vi "Measurement Logic.vi"() -> ()   [LabVIEW 2021, in "Crosstalk Sweep.lvlib"]
uses:
  Crosstalk Sweep.lvlib
  Measurement Configuration.ctl
  shared/controls/digital output level units.ctl
  shared/controls/sweep profile.ctl
  shared/controls/weighting filter.ctl
  shared/controls/highpass filter.ctl
  shared/controls/lowpass filter.ctl
  Measurement Results.ctl
  <vilib>/MeasurementLink/MeasurementLink Measurement Server/Measure Call Context/Measure Call Context.lvclass
  shared/controls/audio filter settings.ctl
  <vilib>/Analysis/1siggen.llb/Ramp Pattern by Samples.vi
  <vilib>/addons/_NISVFA/_Shared subVIs/Common/SVL Set dB Reference (N Ch - 1 Ref).vi
  <vilib>/addons/_NISVFA/_Spectrum Processing/SVFA Unit Conversion (Complex) (N Ch).vi
  <vilib>/addons/_NISVFA/_Spectrum Processing/SVFA Unit Conversion (Complex) (1 Ch).vi
  <vilib>/addons/_NISVFA/_Shared subVIs/Common/SVL Set dB Reference (1 Ch).vi
  <vilib>/addons/_NISVFA/_Shared subVIs/Common/svc_Log View for Spectrum (1Ch).vi
  <vilib>/addons/_NISVFA/_Spectrum Processing/SVFA Unit Conversion (1 Ch).vi
  <vilib>/addons/_NISVFA/_Shared subVIs/Common/svc_Complex Datatype Defaults.vi
  <vilib>/addons/_NISVFA/_Shared subVIs/Common/SVL Set dB Reference (variant).vi
  <vilib>/addons/_NISVFA/_Shared subVIs/Common/svc_Unwrap Phase.vi
  <vilib>/addons/_NISVFA/_Shared subVIs/Common/svc_Convert Spectrum Array to dB.vi
  <vilib>/addons/_NISVFA/_Shared subVIs/Common/svc_Spectrum Units.vi
  <vilib>/addons/_NISVFA/_Spectrum Processing/subVIs/svfa_Conversion Utility (spectrum info).vi
  <vilib>/addons/_NISVFA/_Shared subVIs/Common/svc_Format Value (DBL).vi
  <vilib>/addons/_NISVFA/_Shared subVIs/Common/svc_Get Weighting Enum and Labels.vi
  <vilib>/addons/_NISVFA/_Shared subVIs/Common/svc_Engineering Units to Unit Label.vi
  <vilib>/addons/_NISVFA/_Shared subVIs/Common/svc_Surround NonAlpha String with Parentheses.vi
  <vilib>/dlg_ctls.llb/Space Constant.vi
  <vilib>/addons/_NISVFA/_Spectrum Processing/subVIs/svfa_Peak to RMS to Peak2Peak.vi
  <vilib>/addons/_NISVFA/_Spectrum Processing/subVIs/svfa_Mag to Mag2.vi
  <vilib>/addons/_NISVFA/_Spectrum Processing/subVIs/svfa_Linear to dB.vi
  <vilib>/addons/_NISVFA/_Spectrum Processing/subVIs/svfa_dBrefA to dBrefB.vi
  <vilib>/addons/_NISVFA/_Spectrum Processing/subVIs/svfa_Spectrum to Spectral Density.vi
  <vilib>/addons/_NISVFA/_Shared subVIs/Common/svc_Unit Label Lexical Class.vi
  <vilib>/addons/_NISVFA/_Shared subVIs/Common/svc_Window Parameters.vi
  <vilib>/DAQmx/create/channels.llb/DAQmx Create Channel (AI-Voltage-Basic).vi
  <vilib>/DAQmx/configure/timing.llb/DAQmx Timing (Sample Clock).vi
  <vilib>/Waveform/WDTOps.llb/WDT Get Waveform Subset DBL.vi
  <vilib>/addons/_NISVFA/_Shared subVIs/Common/svc_Caller VI Returned in Error Source.vi
  <vilib>/Analysis/4window.llb/window parameters.vi
  <vilib>/Analysis/4window.llb/Window Properties.vi
  <vilib>/Analysis/4window.llb/Window Properties by Name.vi
  <vilib>/Analysis/NI_AALBase.lvlib
  shared/digital serial api/Digital Serial.lvclass
  shared/digital serial gen settings/digital audio protocol controls.lvlib
  shared/controls/audio controls.lvlib
panel:
  out "XY Graph":cluster{"X data":dbl[], "Y data":dbl[]}[](graph)=[{"X data"=[1000.0000079066498, 1444.4445068435625, 1888.8885404873877, 2333.332974551163, 2777.7776191924368, 3222.2221837594147, 3666.6669921625667, 4111.111180056958, 4555.555303242544, 5000.000080001889], "Y data"=[-83.02077381288392, -79.93403033517882, -79.67645242718531, -75.93201157658373, -75.45566870671045, -74.17335893170335, -72.78173878108285, -72.07408908843989, -70.96339966107612, -70.06311639272025]}, {"X data"=[1000.0000079066498, 1444.4445068435625, 1888.8885404873877, 2333.332974551163, 2777.7776191924368, 3222.2221837594147, 3666.6669921625667, 4111.111180056958, 4555.555303242544, 5000.000080001889], "Y data"=[-100.3560709729349, -100.71622632785073, -100.77370759881723, -100.70292296094586, -100.93312934835308, -99.69443859013792, -100.53907016781393, -100.4790465149002, -101.0239883463542, -100.13211237211175]}, {"X data"=[1000.0000079066498, 1444.4445068435625, 1888.8885404873877, 2333.332974551163, 2777.7776191924368, 3222.2221837594147, 3666.6669921625667, 4111.111180056958, 4555.555303242544, 5000.000080001889], "Y data"=[-117.76654421705797, -127.52260822953843, -128.9925376198278, -120.72766654102435, -118.4793948341033, -122.29285627461928, -135.7344906838366, -121.41325998155511, -120.01195459277108, -131.15607832666257]}]
  out "Spectrum":cluster{"x0":dbl, "dx":dbl, "magnitude":dbl[]}[](graph)
  out "Waveform Graph":waveform(dbl)[](graph)
  out "measure call context out":refnum<class "Measure Call Context.lvclass">
  in  "measure call context in":refnum<class "Measure Call Context.lvclass">
  out "measurement results":T1={"channel names"=["PXI1Slot4/ai0", "PXI1Slot4/ai1", "PXI1Slot2/ai0", "PXI1Slot2/ai1"], "frequency (Hz)"=[1000.0000079066498, 1444.4445068435625, 1888.8885404873877, 2333.332974551163, 2777.7776191924368, 3222.2221837594147, 3666.6669921625667, 4111.111180056958, 4555.555303242544, 5000.000080001889], "crosstalk (dB)"=[-83.02077381288392, -79.93403033517882, -79.67645242718531, -75.93201157658373, -75.45566870671045, -74.17335893170335, -72.78173878108285, -72.07408908843989, -70.96339966107612, -70.06311639272025, -100.3560709729349, -100.71622632785073, -100.77370759881723, -100.70292296094586, -100.93312934835308, -99.69443859013792, -100.53907016781393, -100.4790465149002, -101.0239883463542, -100.13211237211175, -117.76654421705797, -127.52260822953843, -128.9925376198278, -120.72766654102435, -118.4793948341033, -122.29285627461928, -135.7344906838366, -121.41325998155511, -120.01195459277108, -131.15607832666257], "wfm - t0"=0.0, "wfm - dt"=1.9531249997269942e-05, "wfm - data"=array[20480 elements], "fft - f0"=0.0, "fft - df"=10.00000000139779, "fft - data"=array[10240 elements]}
  in  "measurement configuration":T2={"digital serial cfg file"="C:\\Users\\SEBUADV\\Desktop\\Jack\\TAS6424.dsgcfg", "digital channel list"="7821\\PCMo 8", "master clock channel list"="7821\\PCMo 0", "digital audio interferrer channel"=0, "output level"=10.0, "output level units"=enum."% FS", "output range (pk-pk)"=15.0, "load impedance"=4.0, "acq channel - victim"="PXI1Slot4/ai1, PXI1Slot2/ai0:1", "acq channel - interferrer"="PXI1Slot4/ai0", "acq sampling rate"=51200.0, "sweep start frequency (Hz)"=1000.0, "sweep stop frequency (Hz)"=5000.0, "number of steps"=10, "sweep profile"=enum."Linear", "min measurement cycles"=20, "min measurement time (s)"=0.1, "min settling cycles"=0, "min settling time (s)"=0.005, "weighting filter"=enum."Linear", "highpass filter"=enum."DC", "lowpass filter"=enum."No filter"} {"min measurement time (s)" format="%0.2f"; "acq sampling rate" format="%0.2f"}
  out "error out":errorcluster
  in  "error in":errorcluster
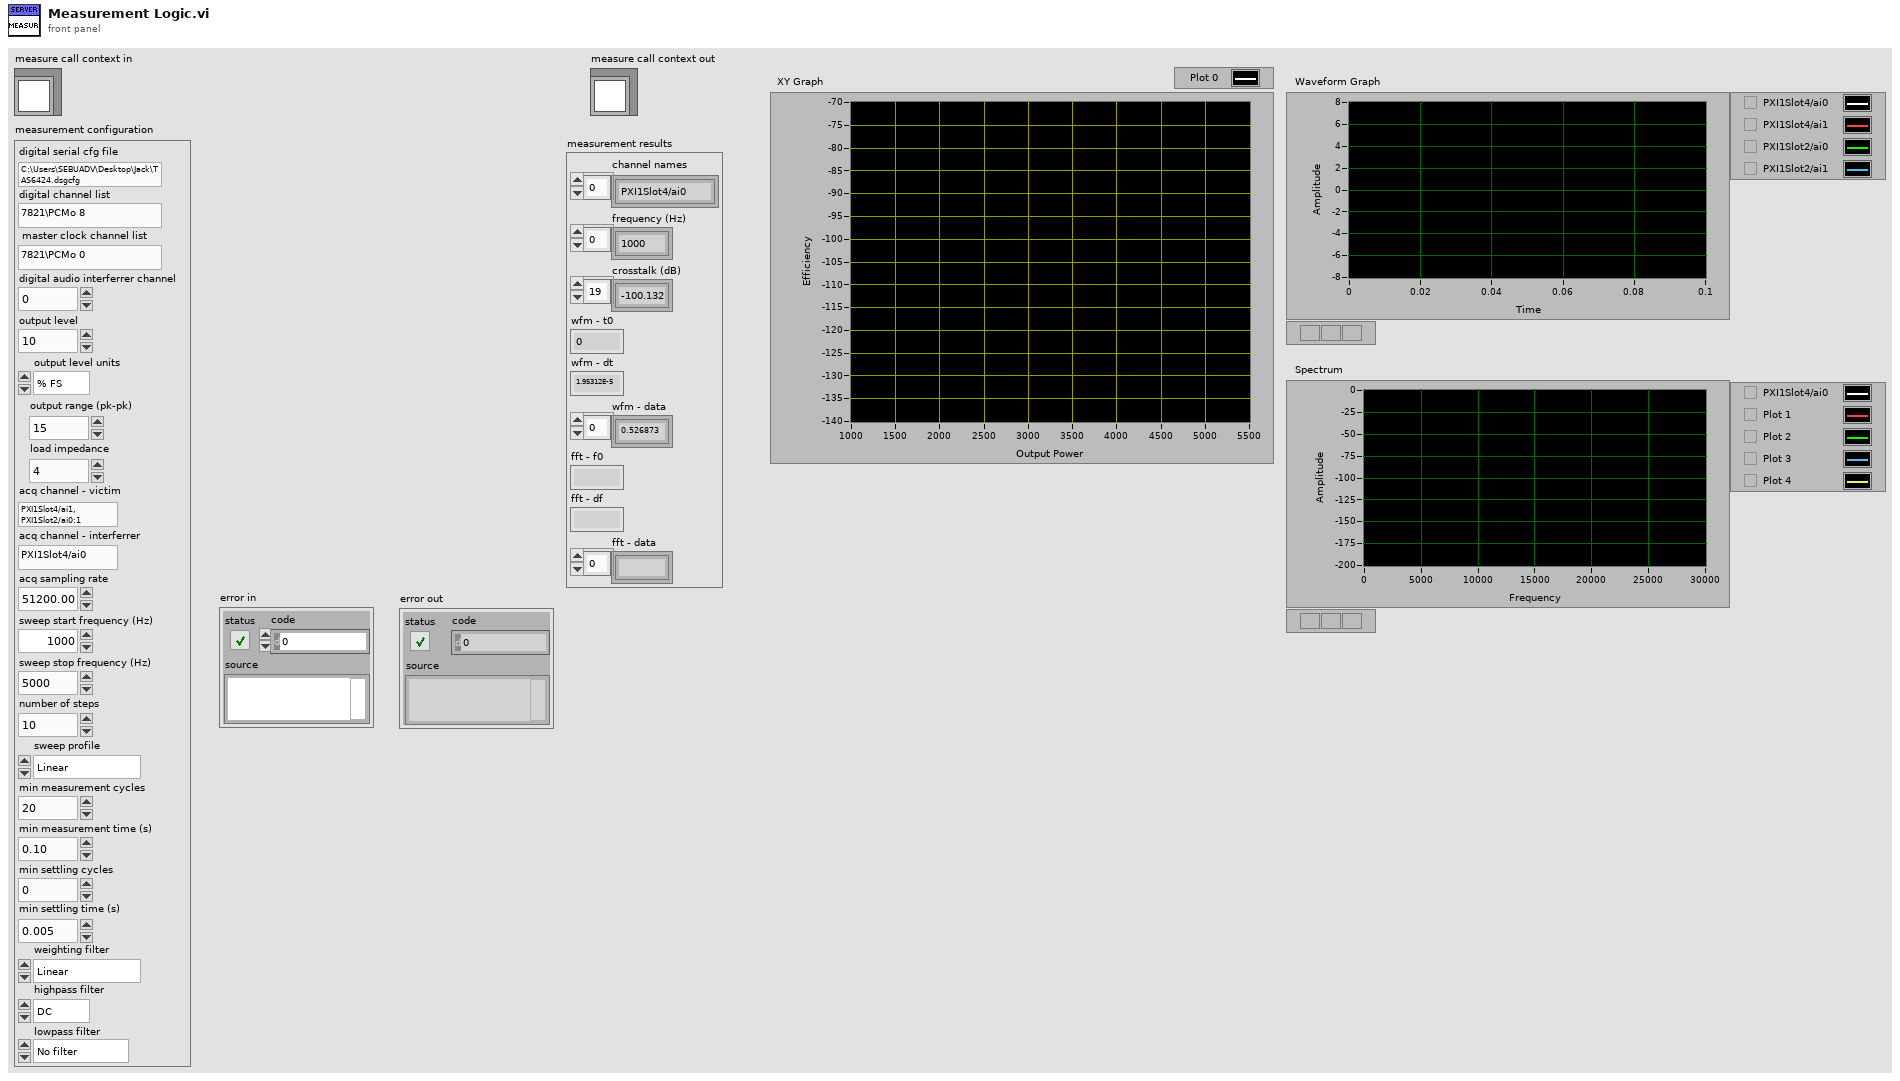
[diagram p1: front panel]
types:
  T1 = typedef "Crosstalk Sweep.lvlib/Measurement Results.ctl" = cluster{"channel names":string[], "frequency (Hz)":dbl[], "crosstalk (dB)":dbl[], "wfm - t0":dbl, "wfm - dt":dbl, "wfm - data":dbl[], "fft - f0":dbl, "fft - df":dbl, "fft - data":dbl[]}
  T2 = typedef "Crosstalk Sweep.lvlib/Measurement Configuration.ctl" = cluster{"digital serial cfg file":string, "digital channel list":string, "master clock channel list":string, "digital audio interferrer channel":i32, "output level":dbl, "output level units":T3, "output range (pk-pk)":dbl, "load impedance":dbl, "acq channel - victim":string, "acq channel - interferrer":string, "acq sampling rate":dbl, "sweep start frequency (Hz)":dbl, "sweep stop frequency (Hz)":dbl, "number of steps":u32, "sweep profile":T4, "min measurement cycles":u32, "min measurement time (s)":dbl, "min settling cycles":u32, "min settling time (s)":dbl, "weighting filter":T5, "highpass filter":T6, "lowpass filter":T7}
  T3 = typedef "audio controls.lvlib/digital output level units.ctl" = enum32{"% FS", "dBFS", "V"}
  T4 = typedef "audio controls.lvlib/sweep profile.ctl" = enum32{"Linear", "Logarithmic"}
  T5 = typedef "weighting filter.ctl" = enum32{"Linear", "A-weighting", "B-weighting", "C-weighting"}
  T6 = typedef "highpass filter.ctl" = enum32{"DC", "AC"}
  T7 = typedef "lowpass filter.ctl" = enum32{"No filter", "AES17 20kHz", "AES17 40kHz"}
  T8 = typedef "audio filter settings.ctl" = cluster{"weighting filter":T5, "highpass filter":T6, "lowpass filter ":T7}
  T9 = typedef "digital serial gen settings.ctl" = cluster{"number of channels":u32, "data justification":T10, "endianness":T11, "channel length":u32, "bit depth":u32, "frame clock rate":dbl, "bit clock edge sync":T12, "master clock rate":dbl, "Logic Level":T13, "frame sync edge for channel 0":T12, "Channel 0 Offset":u32}
  T10 = typedef "PDM Shared.lvlib/PCM Data Justification.ctl" = enum16{"Left Justified", "Right Justified"}
  T11 = typedef "PDM Shared.lvlib/PCM Bit Endianness.ctl" = enum16{"MSB First", "LSB First"}
  T12 = typedef "PDM Shared.lvlib/Digital Edge.ctl" = enum8{"Rising", "Falling"}
  T13 = typedef "PDM Acquisition Class Library.lvlib/DecoderSession.lvclass/Logic Levels.ctl" = enum16{"3.3 V", "1.8 V", "1.2 V"}
  T14 = typedef "AudioGenTypeDefs.lvlib/digital protocol settings.ctl" = cluster{"logic level":T13, "PCM Data Configuration":T15, "bit clock rate":sgl, "master clock rate":sgl, "clock mode":T16, "Frame Sync Clock Control":T17}
  T15 = typedef "PDM Shared.lvlib/PCM Data Format Configuration.ctl" = cluster{"Frame Sync Edge for Channel 0":T12, "Channel Count Per Frame":u8, "Channel Length":u16, "Bit Depth":u8, "Channel 0 Offset":u16, "Endianness":T11, "Data Justification":T10}
  T16 = typedef "PDM Shared.lvlib/clock mode.ctl" = enum16{"divided clock", "DDS"}
  T17 = typedef "PDM Shared.lvlib/PCM Frame Sync Control.ctl" = cluster{"Frame Length":u16, "Frame Sync Pulse Width":u16, "Bit Clock Edge  Sync":T12}
  T18 = cluster{"frequency":dbl, "amplitude":dbl, "phase":dbl}[]
  T19 = cluster{"linear/dB":enum16{"no change", "linear", "dB"}, "dB reference (0: no change)":dbl, "power/magnitude":enum16{"no change", "power", "magnitude"}, "view":enum16{"no change", "rms", "peak", "peak-peak"}}
  T20 = typedef "svc_Spectrum Info.ctl" = cluster{"channel name":string, "description":string, "x-axis units":T21, "spectral info":cluster{"spectrum type":T22, "linear/dB":enum16{"linear", "dB"}, "window":u16, "window size":i32, "FFT size":i32}, "engineering units":T23, "custom label":string, "dB reference [EU]":dbl, "peak units":enum16{"rms", "peak", "peak-peak"}, "weighting filter":T24, "spectral density?":bool, "unit label":string, "spectrum skewed?":bool, "complimentary spectrum units":T25}
  T21 = typedef "svc_X-Axis Units.ctl" = u16
  T22 = typedef "svc_Spectrum Type.ctl" = enum16{"FFT Spectrum [complex]", "Amplitude [Magnitude]", "Power [Magnitude^2]", "Cross Spectrum [complex]", "Frequency Response [Complex]"}
  T23 = typedef "svc_Engineering Units Text Ring.ctl" = u16
  T24 = typedef "svc_Weighting Filter Text Ring.ctl" = u16
  T25 = typedef "svc_Complimentary Spectrum Units.ctl" = enum16{"none", "radians", "degrees", "cycles", "imaginary"}
  T26 = cluster{"complex spectrum response":cluster{"f0":dbl, "df":dbl, "complex spectrum":cdb[]}, "spectrum info":T20}
  T27 = cluster{"complex spectrum response":cluster{"f0":dbl, "df":dbl, "complex spectrum":cdb[]}, "spectrum info":T20}[]
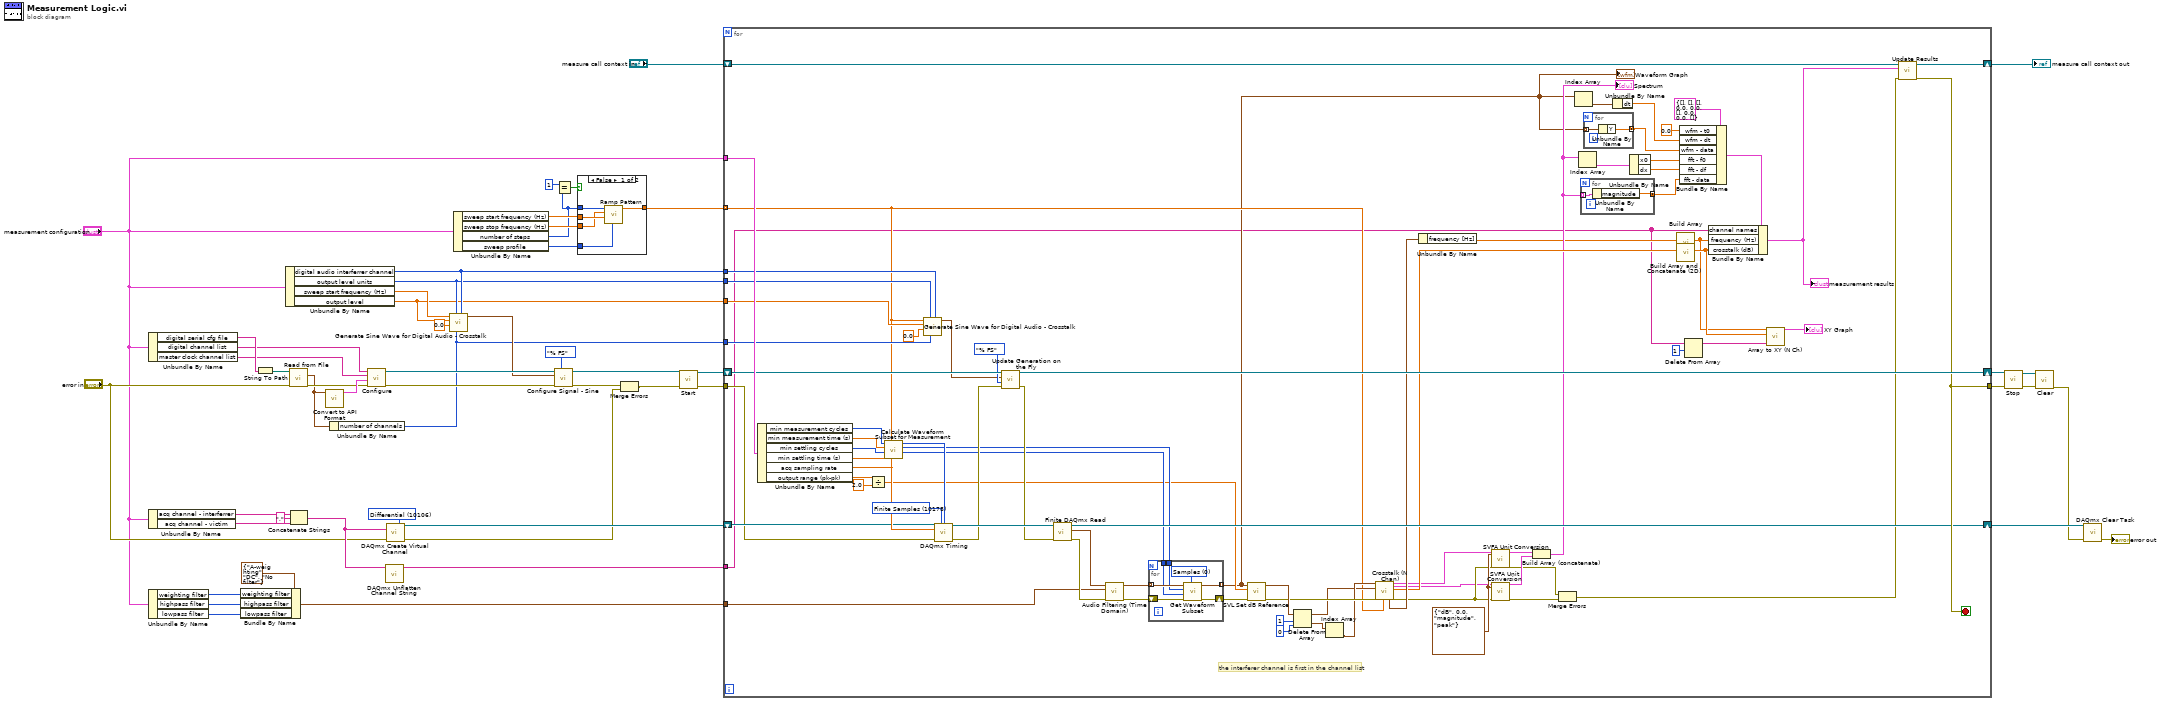
[diagram p0: block diagram]
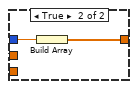
[diagram p2: hidden frame]
diagram:
  w28 = 10106 items=["Default"=-1, "RSE"=10083, "NRSE"=10078, "Differential"=10106, "Pseudodifferential"=12529] ("input terminal configuration")
  n1 = Unbundle By Name("measurement configuration") -> ("digital serial cfg file"=w44:string, "digital channel list"=w40:string, "master clock channel list"=w39:string)
  n2 = Unbundle By Name("measurement configuration") -> ("acq channel - interferrer"=w27:string, "acq channel - victim"=w26:string)
  n3 = Unbundle By Name("measurement configuration") -> ("weighting filter"=w4:T5, "highpass filter"=w3:T6, "lowpass filter"=w2:T7)
  n4 = Bundle By Name(cluster=T8 {"weighting filter"=enum."A-weighting", "highpass filter"=enum."DC", "lowpass filter "=enum."No filter"} ("filter settings"), "weighting filter"=w4, "highpass filter"=w3, "lowpass filter"=w2) -> (w1:T8)
  n5 = String To Path(string=w44) -> (path=w41:path)
  n6 = Unbundle By Name("measurement configuration") -> ("digital audio interferrer channel"=w17:i32, "output level units"=w16:T3, "sweep start frequency (Hz)"=w31:dbl, "output level"=w15:dbl)
  n7 = call "Read from File.vi"("error in (no error)"="error in", "file path"=w41) -> ("error out"=w42:errorcluster, "digital audio protocol settings"=w33:T9)  [unwired: 7 in, 1 out]
  n8 = Concatenate Strings(w27, "," ("string"), w26) -> (w24:string)
  n9 = call "Convert to API Format.vi"("digital audio protocol settings"=w33) -> ("digital protocol settings"=w43:T14)  [unwired: 10 in]
  n10 = Unbundle By Name(w33) -> ("number of channels"=w14:u32)
  n11 = call "Configure.vi"("error in (no error)"=w42, "digital protocol settings"=w43, "master clock channel list"=w39, "data channel list"=w40) -> ("error out"=w38:errorcluster, "digital serial task"=w37:refnum<class "Digital Serial.lvclass">)  [unwired: 6 in]
  n12 = call <vilib>:"DAQmx Unflatten Channel String.vi"("names in"=w24) -> ("names out"=w18:string[])  [unwired: 13 in, 1 out]
  n13 = call-poly <vilib>:"DAQmx Create Virtual Channel.vi"("input terminal configuration"=w28, "physical channels"=w24, "error in"="error in") -> ("task out"=w20:refnum<k21>, "error out"=w19:errorcluster)  [unwired: 11 in]
  n14 = call "Generate Sine Wave for Digital Audio - Crosstalk.vi"("interferrer channel"=w17, "number of channels"=w14, "output level units"=w16, "phase"=0.0, "amplitude"=w15, "frequency"=w31) -> ("signals"=w32:T18)  [unwired: 5 in]
  n15 = Unbundle By Name("measurement configuration") -> ("sweep start frequency (Hz)"=w50:dbl, "sweep stop frequency (Hz)"=w49:dbl, "number of steps"=w47:u32, "sweep profile"=w51:T4)
  n16 = call "Configure Signal - Sine.vi"("output level units"=digital_output_level_units."% FS", "error in (no error)"=w38, "sine wave properties"=w32, "Digital Serial in"=w37) -> ("error out"=w35:errorcluster, "Digital Serial out"=w36:refnum<class "Digital Serial.lvclass">)  [unwired: 6 in]
  n17 = Equal?(x=u32 1, y=w47) -> (x = y?=w48:bool)
  n18 = case shown="False" w48 {
    tunnel: w51 -> [w58 _]
    tunnel: w50 -> [w57 w60]
    tunnel: w49 -> [w56 _]
    tunnel: w47 -> [w55 _]
    tunnel: [w54 w59] -> w45
    frame False {
      n19 = call-poly <vilib>:"Ramp Pattern.vi"("type"=w58, "start"=w57, "end"=w56, "samples"=w55) -> ("Ramp Pattern"=w54:dbl[])  [unwired: 6 in, 1 out]
    }
    frame True {
      n20 = Build Array(w60) -> (w59:dbl[])
    }
  }
  n21 = Merge Errors(w35, w19) -> (w34:errorcluster)
  n22 = call "Start.vi"("error in (no error)"=w34, "Digital Serial in"=w36) -> ("error out"=w21:errorcluster, "Digital Serial out"=w22:refnum<class "Digital Serial.lvclass">)  [unwired: 8 in]
  n23 = for {
    tunnel: w45 -> [w86] mode=indexing
    shift-right: [w136] -> w53
    shift-left: "measure call context in" -> [w135]
    shift-right: [w105] -> w9
    shift-left: w20 -> [w121]
    shift-right: [w107] -> w11
    shift-left: w22 -> [w116]
    tunnel: w21 -> [w120]
    tunnel: "measurement configuration" -> [w119]
    tunnel: w18 -> [w64]
    tunnel: w17 -> [w114]
    tunnel: w16 -> [w113]
    tunnel: w15 -> [w111]
    tunnel: w14 -> [w110]
    tunnel: [w106] -> w10
    tunnel: w1 -> [w100]
    stop <- w106 stop-if-true
    w83 = T19 {"linear/dB"=enum."dB", "dB reference (0: no change)"=0.0, "power/magnitude"=enum."magnitude", "view"=enum."peak"} ("desired scaling")
    w123 = 10178 items=["Finite Samples"=10178, "Continuous Samples"=10123, "Hardware Timed Single Point"=12522] ("sample mode")
    # "the interferer channel is first in the channel list"
    n24 = Unbundle By Name(w119) -> ("min measurement cycles"=w128:u32, "min measurement time (s)"=w127:dbl, "min settling cycles"=w126:u32, "min settling time (s)"=w125:dbl, "acq sampling rate"=w122:dbl, "output range (pk-pk)"=w95:dbl)
    n25 = Divide(x=w95, y=2.0) -> (x/y=w94:dbl)
    n26 = call "Calculate Waveform Subset for Measurement.vi"("sampling rate"=w122, "signal frequency"=w86, "minimum settling duration"=w125, "minimum settling cycles"=w126, "minimum measurement duration"=w127, "minimum measurement cycles"=w128) -> ("duration (samples)"=w98:u32, "start (samples)"=w99:u32, "total acquisition (samples)"=w124:u32)  [unwired: 3 in]
    n27 = call "Generate Sine Wave for Digital Audio - Crosstalk.vi"("interferrer channel"=w114, "number of channels"=w110, "output level units"=w113, "phase"=0.0, "amplitude"=w111, "frequency"=w86) -> ("signals"=w109:T18)  [unwired: 5 in]
    n28 = call-poly <vilib>:"DAQmx Timing.vi"("task/channels in"=w121, "sample mode"=w123, "samples per channel"=w124, "rate"=w122, "error in"=w120) -> ("task out"=w118:refnum<k21>, "error out"=w117:errorcluster)  [unwired: 9 in]
    n29 = call "Update Generation on the Fly.vi"("error in (no error)"=w117, "output level units"=digital_output_level_units."% FS", "sine wave properties"=w109, "Digital Serial in"=w116) -> ("error out"=w108:errorcluster, "Digital Serial out"=w107:refnum<class "Digital Serial.lvclass">)  [unwired: 6 in]
    n30 = call "Finite DAQmx Read.vi"("error in (no error)"=w108, "task/channels in"=w118) -> ("error out"=w101:errorcluster, "data"=w102:waveform(dbl)[], "task out"=w105:refnum<k21>)  [unwired: 7 in]
    n31 = call "Audio Filtering (Time Domain).vi"("waveforms"=w102, "filter settings"=w100, "error in"=w101) -> ("time domain"=w103:waveform(dbl)[], "error out"=w104:errorcluster)  [unwired: 6 in]
    n32 = for {
      tunnel: w103 -> [w143] mode=indexing
      tunnel: [w142] -> w69 mode=indexing
      shift-right: [w139] -> w97
      shift-left: w104 -> [w140]
      tunnel: w99 -> [w138]
      tunnel: w98 -> [w137]
      w141 = u16 0 items=["Samples", "Relative Time"] ("start/duration format")
      n33 = call-poly <vilib>:"Get Waveform Subset.vi"("start/duration format"=w141, "error in (no error)"=w140, "duration"=w137, "start samples/time"=w138, "waveform in"=w143) -> ("error out"=w139:errorcluster, "waveform out"=w142:waveform(dbl))  [unwired: 1 in, 2 out]
    }
    "Waveform Graph" <- w69
    n34 = call-poly <vilib>:"SVL Set dB Reference.vi"("error in (no error)"=w97, "dB reference [EU]"=w94, "scaled signals in [EU]"=w69) -> ("error out"=w89:errorcluster, "scaled signals out [EU]"=w90:waveform(dbl)[])  [unwired: 7 in]
    n35 = Delete From Array(array=w90, length=1, index=0) -> (deleted portion=w91:waveform(dbl)[], array with subset deleted=w87:waveform(dbl)[])
    n36 = Index Array(array=w91) -> (element=w88:waveform(dbl))  [unwired: 1 in]
    n37 = call "Crosstalk (N Chan).vi"("stimulus signal"=w88, "idle channel response"=w87, "error in (no error)"=w89, "expected fundamental frequency [Hz]"=w86) -> ("detected tone stimulus"=w85:cluster{"frequency [Hz]":dbl, "amplitude":dbl}, "complex spectrum\nstimulus X"=w79:T26, "complex spectrum idle-channel response"=w80:T27, "crosstalk"=w84:dbl[], "error out"=w81:errorcluster)  [unwired: 8 in, 3 out]
    n38 = Unbundle By Name(w85) -> ("frequency [Hz]"=w68:dbl)
    n39 = call-poly <vilib>:"SVFA Unit Conversion.vi"("complex spectrum"=w79, "desired scaling"=w83, "error in (no error)"=w81) -> ("converted spectrum"=w61:cluster{"x0":dbl, "dx":dbl, "magnitude":dbl[]}, "error out"=w77:errorcluster)  [unwired: 11 in, 4 out]
    n40 = call-poly <vilib>:"SVFA Unit Conversion.vi"("complex spectra"=w80, "desired scaling"=w83, "error in (no error)"=w81) -> ("converted spectra"=w82:cluster{"x0":dbl, "dx":dbl, "magnitude":dbl[]}[], "error out"=w78:errorcluster)  [unwired: 11 in, 4 out]
    n41 = Build Array (concatenate)(w61, w82) -> (w72:cluster{"x0":dbl, "dx":dbl, "magnitude":dbl[]}[])
    "Spectrum" <- w72
    n42 = Merge Errors(w77, w78) -> (w76:errorcluster)
    n43 = Index Array(array=w69) -> (element=w71:waveform(dbl))  [unwired: 1 in]
    n44 = Index Array(array=w72) -> (element=w75:cluster{"x0":dbl, "dx":dbl, "magnitude":dbl[]})  [unwired: 1 in]
    n45 = for {
      tunnel: [w145] -> w129 mode=concatenating
      tunnel: w72 -> [w144] mode=indexing
      n46 = Unbundle By Name(w144) -> ("magnitude"=w145:dbl[])
    }
    n47 = for {
      tunnel: [w147] -> w130 mode=concatenating
      tunnel: w69 -> [w146] mode=indexing
      n48 = Unbundle By Name(w146) -> ("Y"=w147:dbl[])
    }
    n49 = Unbundle By Name(w71) -> ("dt"=w70:dbl)
    n50 = Unbundle By Name(w75) -> ("x0"=w74:dbl, "dx"=w73:dbl)
    n51 = call "Build Array.vi"("value"=w68) -> ("Array"=w65:dbl[])  [unwired: 10 in]
    n52 = call "Build Array and Concatenate (2D).vi"("Array"=w84) -> ("Array Out"=w66:dbl[])  [unwired: 10 in]
    n53 = Bundle By Name(cluster=T1 {"channel names"=[], "frequency (Hz)"=[], "crosstalk (dB)"=[], "wfm - t0"=0.0, "wfm - dt"=0.0, "wfm - data"=[], "fft - f0"=0.0, "fft - df"=0.0, "fft - data"=[]} ("Measurement Results"), "wfm - t0"=0.0, "wfm - dt"=w70, "wfm - data"=w130, "fft - f0"=w74, "fft - df"=w73, "fft - data"=w129) -> (w132:T1)
    n54 = Delete From Array(array=w64, length=1) -> (array with subset deleted=w63:string[])  [unwired: 1 in, 1 out]
    n55 = Bundle By Name(cluster=w132, "channel names"=w64, "frequency (Hz)"=w65, "crosstalk (dB)"=w66) -> (w131:T1)
    "measurement results" <- w131
    n56 = call "Array to XY (N Ch).vi"("channel names"=w63, "Y data"=w66, "X data"=w65) -> ("XY plots"=→"XY Graph":cluster{"X data":dbl[], "Y data":dbl[]}[])  [unwired: 8 in]
    n57 = call <vilib>:"Update Results.vi"("error in"=w76, "measurement results"=w131, "measure call context in"=w135) -> ("error out"=w106:errorcluster, "measure call context out"=w136:refnum<class "Measure Call Context.lvclass">)  [unwired: 7 in]
  }
  "measure call context out" <- w53
  n58 = call "Stop.vi"("error in (no error)"=w10, "Digital Serial in"=w11) -> ("error out"=w13:errorcluster, "Digital Serial out"=w12:refnum<class "Digital Serial.lvclass">)  [unwired: 8 in]
  n59 = call "Clear.vi"("error in (no error)"=w13, "Digital Serial in"=w12) -> ("error out"=w8:errorcluster)  [unwired: 9 in]
  n60 = call <vilib>:"DAQmx Clear Task.vi"("task in"=w9, "error in"=w8) -> ("error out"=→"error out":errorcluster)  [unwired: 13 in]
